vi "Percent Difference Calculation.vi"(8 "error in (no error)":errorcluster, 10 "Input from UUT Serial Port Output":string, 11 "Input Value from DMM Measurement":dbl) -> (0 "error out":errorcluster, 3 "Percent Different Calculated":dbl format="%#_3g")   [LabVIEW 2025]
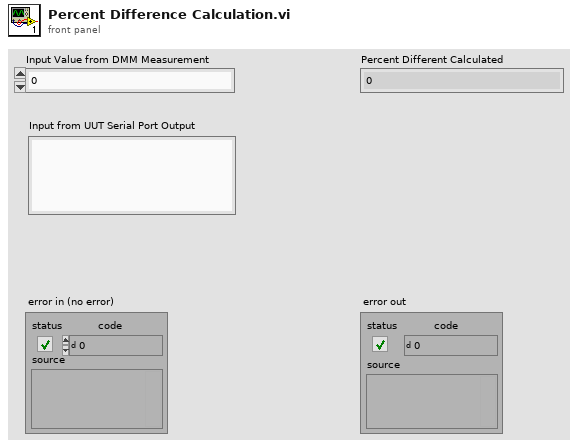
[diagram p1: front panel]
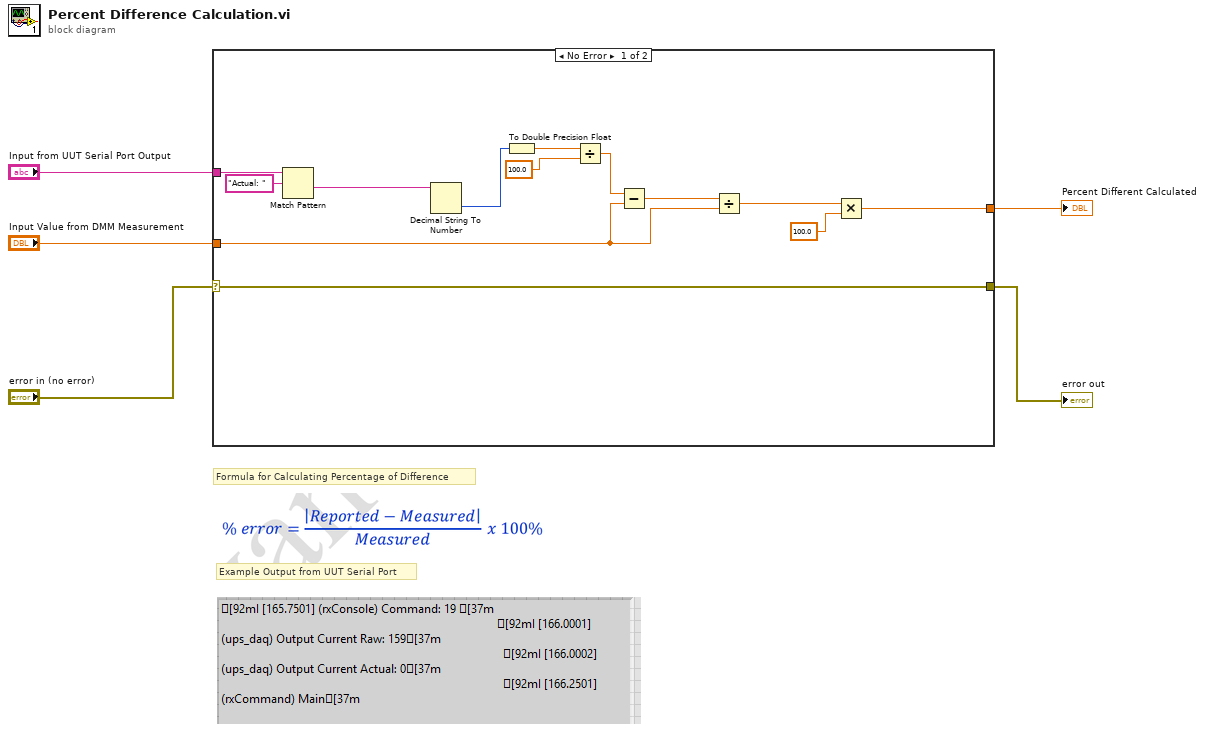
[diagram p0: block diagram]
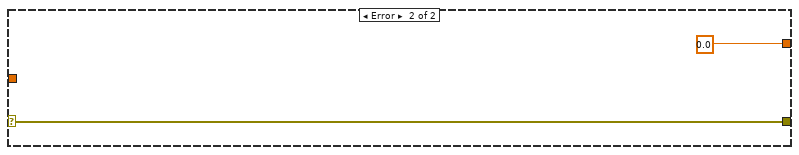
[diagram p2: hidden frame]
diagram:
  # "Example Output from UUT Serial Port"
  # "Formula for Calculating Percentage of Difference"
  n1 = case shown="No Error" "error in (no error)" {
    selector: "error in (no error)" -> [w17 w20]
    tunnel: [w17 w20] -> w4
    tunnel: "Input from UUT Serial Port Output" -> [w15 _]
    tunnel: [w8 0.0] -> w2
    tunnel: "Input Value from DMM Measurement" -> [w9 _]
    frame No Error {
      n2 = Match Pattern(string=w15, regular expression="Actual: ") -> (after substring=w16:string)  [unwired: 1 in, 3 out]
      n3 = Decimal String To Number(string=w16) -> (number=w14:i32)  [unwired: 2 in, 1 out]
      n4 = To Double Precision Float(number=w14) -> (double precision float=w6:dbl)
      n5 = Divide(x=w6, y=100.0) -> (x/y=w11:dbl)
      n6 = Subtract(x=w11, y=w9) -> (x-y=w10:dbl)
      n7 = Divide(x=w10, y=w9) -> (x/y=w12:dbl)
      n8 = Multiply(x=w12, y=100.0) -> (x*y=w8:dbl)
    }
    frame Error {
    }
  }
  "error out" <- w4
  "Percent Different Calculated" <- w2
